vi "Igor_OpenRefnum.vi"(8 "error in (no error)":errorcluster, 11 "Debug Mode? (F)":bool) -> (0 "error out":errorcluster, 3 "Application out":refnum<k7>)   [LabVIEW 2019]
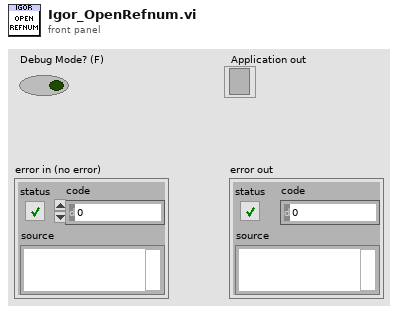
[diagram p1: front panel]
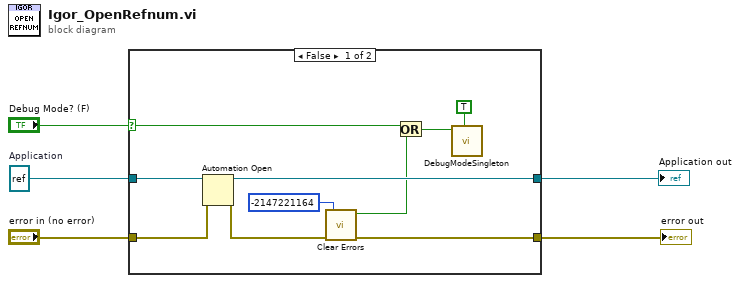
[diagram p0: block diagram]
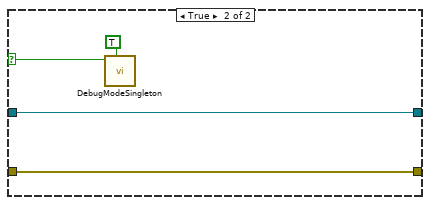
[diagram p2: hidden frame]
diagram:
  w5 = refnum<k7> refnum  # Application
  n1 = case shown="False" "Debug Mode? (F)" {
    selector: "Debug Mode? (F)" -> [w8 w18]
    tunnel: [w10 w16] -> w4
    tunnel: "error in (no error)" -> [w14 w16]
    tunnel: w5 -> [w13 w17]
    tunnel: [w12 w17] -> w3
    frame False {
      n2 = Automation Open(error in (no error)=w14, Automation Refnum=w13) -> (Automation Refnum=w12:refnum<k7>, error out=w11:errorcluster)  [unwired: 2 in]
      n3 = call <vilib>:"Clear Errors.vi"("error in (no error)"=w11, "specific error code to clear (0: all)"=-2147221164) -> ("error out"=w10:errorcluster, "specific error cleared?"=w6:bool)  [unwired: 4 in]
      n4 = Or(x=w8, y=w6) -> (x .or. y?=w7:bool)
      n5 = call "DebugModeSingleton.vi"("Write?"=TRUE, "Debug?"=w7) -> ()  [unwired: 9 in, 1 out]
    }
    frame True {
      n6 = call "DebugModeSingleton.vi"("Write?"=TRUE, "Debug?"=w18) -> ()  [unwired: 9 in, 1 out]
    }
  }
  "error out" <- w4
  "Application out" <- w3
